vi "test fgv net.vi"() -> ()   [LabVIEW 2017]
uses:
  Controls/MQTT FGV Options.ctl
panel:
  out "topicrecieved 2":string
  out "messagereceived 2":string
  in  "Read":bool
  out "Error Info":string
  in  "Message":string
  in  "Topic":string
  in  "Publish":bool
  in  "stop":bool
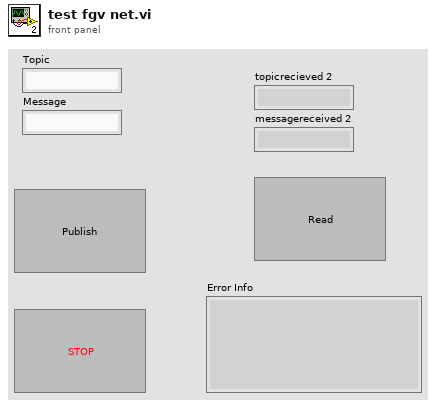
[diagram p1: front panel]
types:
  T1 = typedef "MQTT FGV Options.ctl" = enum16{"Read", "Subscribe", "Publish", "Get Status", "Connect", "Disconnect"}
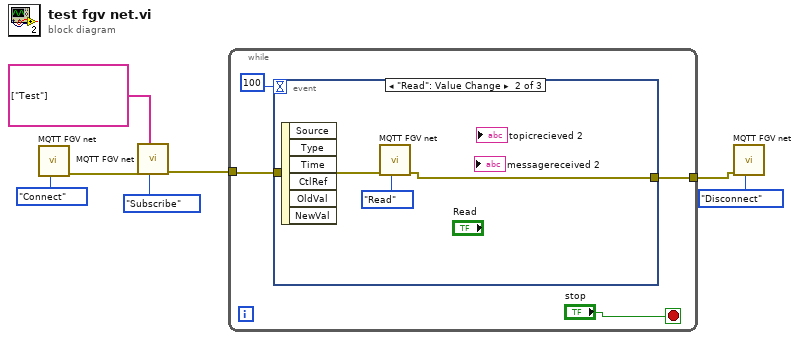
[diagram p0: block diagram]
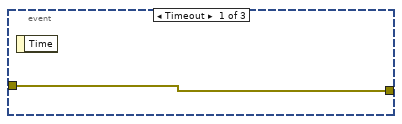
[diagram p2: hidden frame]
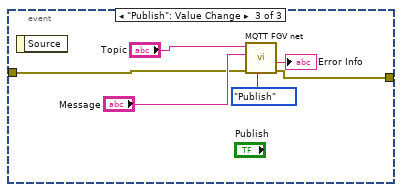
[diagram p3: hidden frame]
diagram:
  n1 = call "MQTT FGV net.vi"("Options"=MQTT_FGV_Options."Connect") -> ("error out"=w2:errorcluster)  [unwired: 6 in, 4 out]
  n2 = call "MQTT FGV net.vi"("Options"=MQTT_FGV_Options."Subscribe", "topics"=string[] ["Test"], "error in (no error)"=w2) -> ("error out"=w5:errorcluster)  [unwired: 4 in, 4 out]
  n3 = while {
    tunnel: w5 -> [w9]
    tunnel: [w8] -> w1
    stop <- "stop" stop-if-true
    n4 = event shown="[1] \"Read\": Value Change" {
      selector: _ -> [_ _ _]
      dyn-events: _ -> [_ _ _]
      timeout: 100 -> [_ _ _]
      tunnel: w9 -> [w12 w14 w18]
      tunnel: [w12 w13 w16] -> w8
      event Timeout {
        n5 = event-data() -> ()  [unwired: 1 in, 1 out]
      }
      event "Read": Value Change {
        n6 = event-data() -> ()  [unwired: 1 in, 6 out]
        n7 = call "MQTT FGV net.vi"("Options"=MQTT_FGV_Options."Read", "error in (no error)"=w14) -> ("error out"=w13:errorcluster)  [unwired: 5 in, 4 out]
      }
      event "Publish": Value Change {
        n8 = event-data() -> ()  [unwired: 1 in, 1 out]
        n9 = call "MQTT FGV net.vi"("Options"=MQTT_FGV_Options."Publish", "error in (no error)"=w18, "Message"="Message", "Topic"="Topic") -> ("error out"=w16:errorcluster, "Error Info"=→"Error Info":string)  [unwired: 3 in, 3 out]
      }
    }
  }
  n10 = call "MQTT FGV net.vi"("Options"=MQTT_FGV_Options."Disconnect", "error in (no error)"=w1) -> ()  [unwired: 5 in, 5 out]
